vi "v2.62.vi"() -> ()   [LabVIEW 2018]
uses:
  <vilib>/DAQmx/read.llb/DAQmx Read (Analog 1D DBL NChan 1Samp).vi
  <extravilib>/ChannelInstances/High Speed Stream-c(a[.](c(dbl,dbl,dbl,dbl)),stamp,a[.](dbl),c(dbl,dbl,dbl,dbl,dbl,dbl,dbl))/_Read For Replicate.vi
  <extravilib>/ChannelInstances/High Speed Stream-c(a[.](c(dbl,dbl,dbl,dbl)),stamp,a[.](dbl),c(dbl,dbl,dbl,dbl,dbl,dbl,dbl))/Instantiate.vi
  <vilib>/Utility/file.llb/Write Delimited Spreadsheet (string).vi
  <extravilib>/ChannelInstances/High Speed Stream-c(a[.](c(dbl,dbl,dbl,dbl)),stamp,a[.](dbl),c(dbl,dbl,dbl,dbl,dbl,dbl,dbl))/)Channel.vi
  <extravilib>/ChannelInstances/High Speed Stream-c(a[.](c(dbl,dbl,dbl,dbl)),stamp,a[.](dbl),c(dbl,dbl,dbl,dbl,dbl,dbl,dbl))/Abort Signal/Init Signal.vi
  <vilib>/DAQmx/create/channels.llb/DAQmx Create Channel (AI-Temperature-Thermocouple).vi
  <vilib>/DAQmx/configure/timing.llb/DAQmx Timing (Sample Clock).vi
  <vilib>/DAQmx/miscellaneous.llb/DAQmx Fill In Error Info.vi
  <extravilib>/ChannelInstances/High Speed Stream-c(a[.](c(dbl,dbl,dbl,dbl)),stamp,a[.](dbl),c(dbl,dbl,dbl,dbl,dbl,dbl,dbl)).lvlib
panel:
  in  "file path (dialog if empty)":path
  out "Enum":T1(ring)
  in  "Start Recording?":bool
  in  "Stop Recording?":bool
  in  "Flowrate Control":dbl
  out "Status":T2(ring)
  in  "OK Button":bool
  in  "DAQ Properties":cluster{"Sample Rate":dbl}={"Sample Rate"=1.0} {"Sample Rate" min=0.1 max=10000.0 step=0.1}
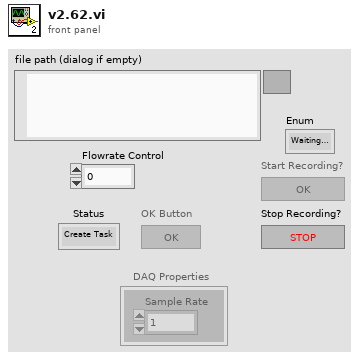
[diagram p1: front panel]
types:
  T1 = enum16{"Waiting to record", "Creating Spreadsheet", "Recording", "Finished Recording"}
  T2 = enum16{"Create Task", "Change Settings", "Check Settings", "Read Data", "End Task"}
  T3 = enum8{"Enabled", "Disabled", "Disabled and Grayed Out"}
  T4 = cluster{"Flowrate Data":cluster{"Line Number":dbl, "Temperature":dbl, "Pressure":dbl, "Flowrate":dbl}[], "Current Time":timestamp, "DAQmx Data":dbl[], "Rig Temperatures":cluster{"BRNR FC":dbl, "BRNR Nozzle":dbl, "Lance Tip":dbl, "Tube 2 Tmp":dbl, "Tube Tmp":dbl, "GA GAS Tmp":dbl, "Chamber External Temp":dbl}}
  T5 = cluster{"BRNR FC":dbl, "BRNR Nozzle":dbl, "Lance Tip":dbl, "Tube 2 Tmp":dbl, "Tube Tmp":dbl, "GA GAS Tmp":dbl, "Chamber External Temp":dbl}
  T6 = cluster{"Line Number":dbl, "Temperature":dbl, "Pressure":dbl, "Flowrate":dbl}[]
  T7 = typedef "High Speed Stream-c(a[.](c(dbl,dbl,dbl,dbl)),stamp,a[.](dbl),c(dbl,dbl,dbl,dbl,dbl,dbl,dbl)).lvlib/)Channel.ctl" = refnum<queue>
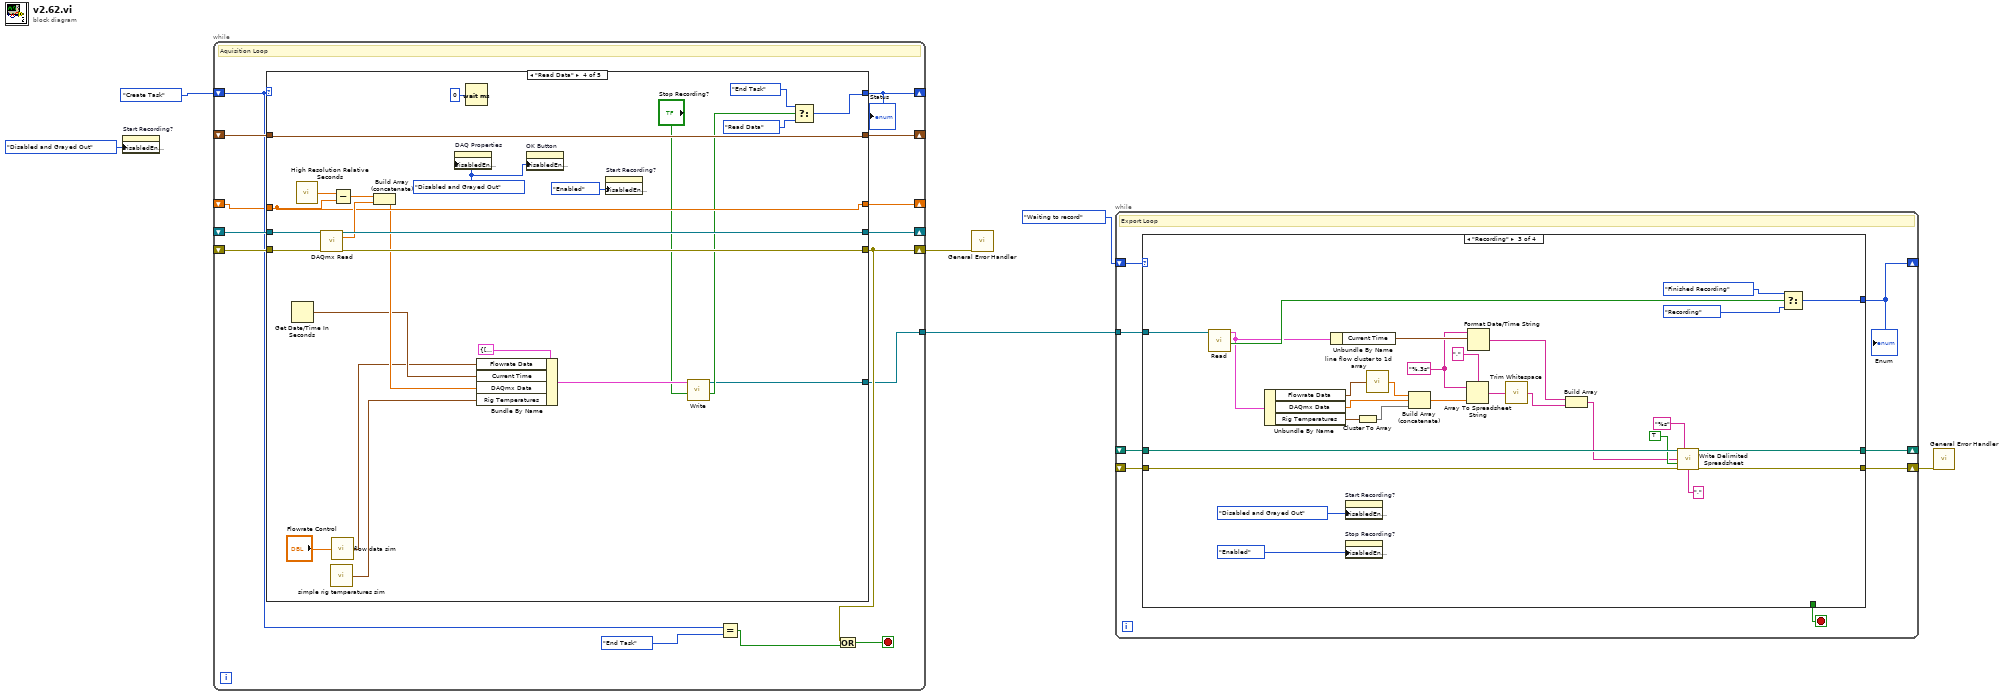
[diagram p0: block diagram]
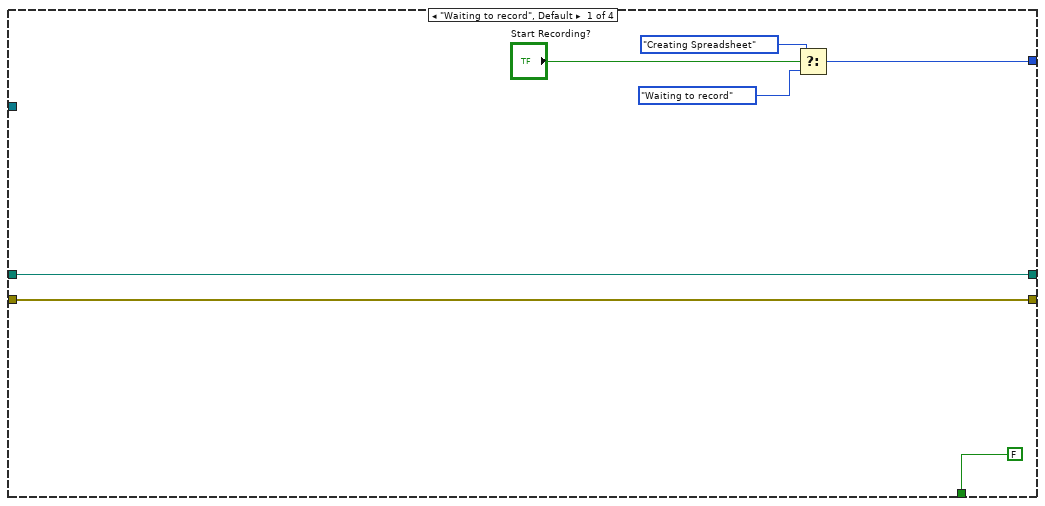
[diagram p2: hidden frame]
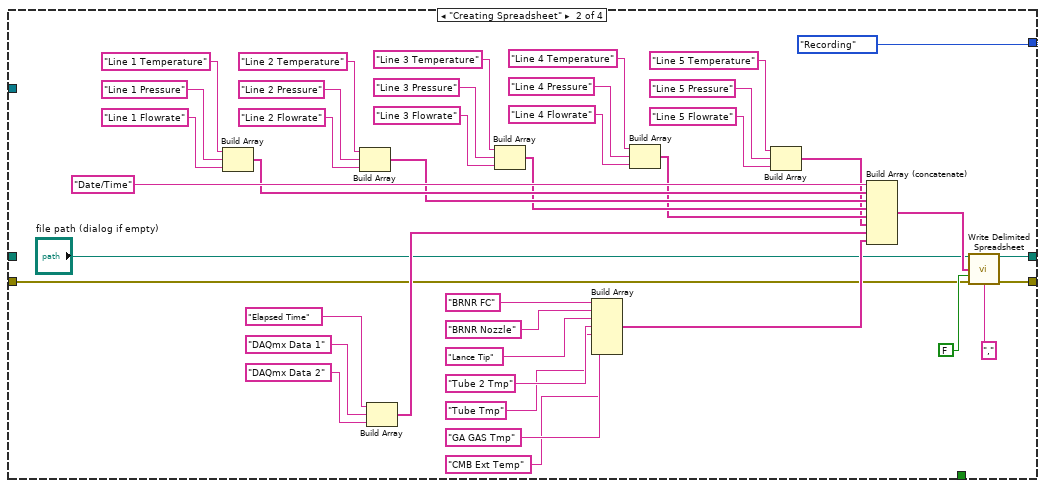
[diagram p3: hidden frame]
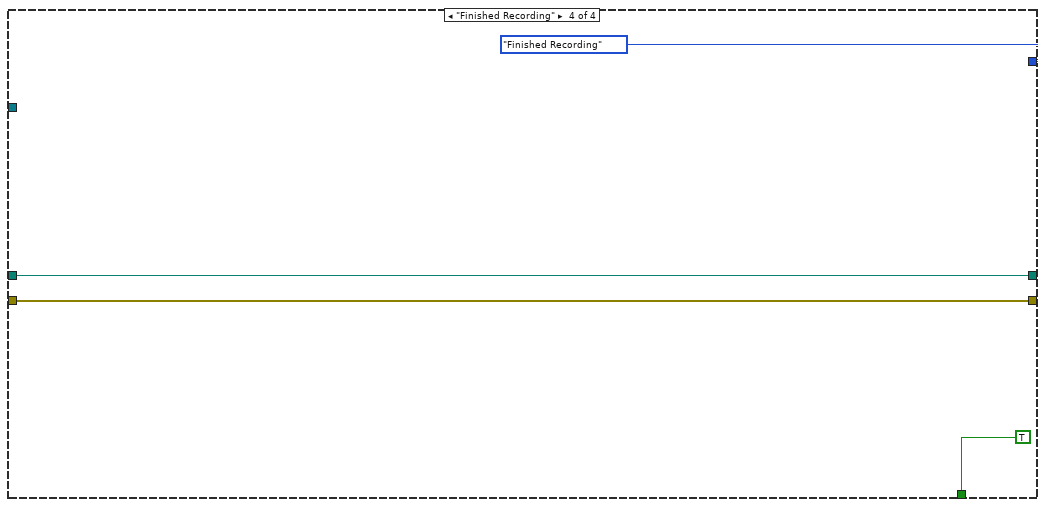
[diagram p4: hidden frame]
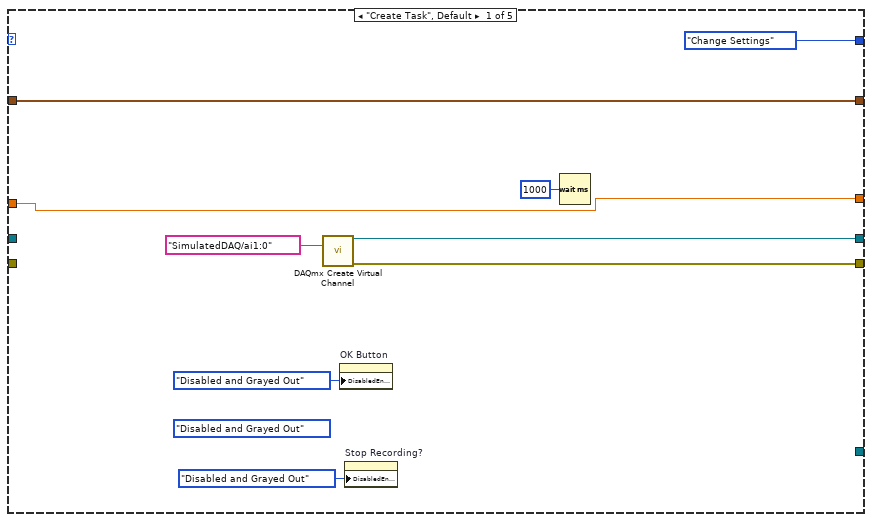
[diagram p5: hidden frame]
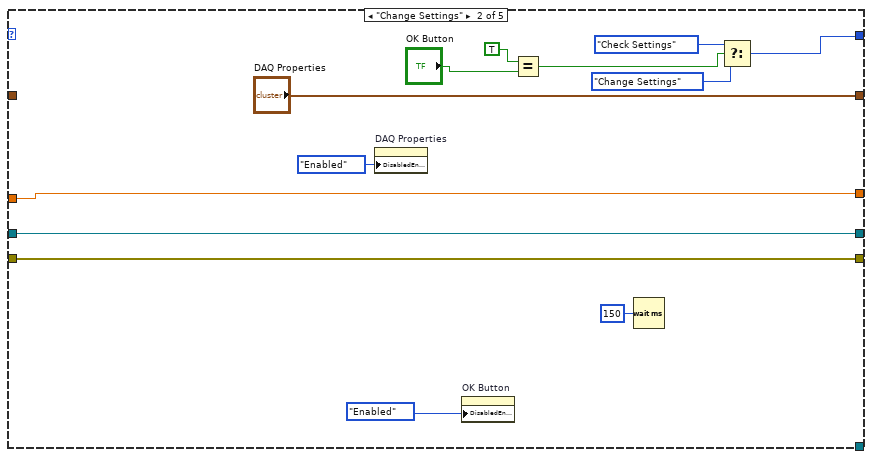
[diagram p6: hidden frame]
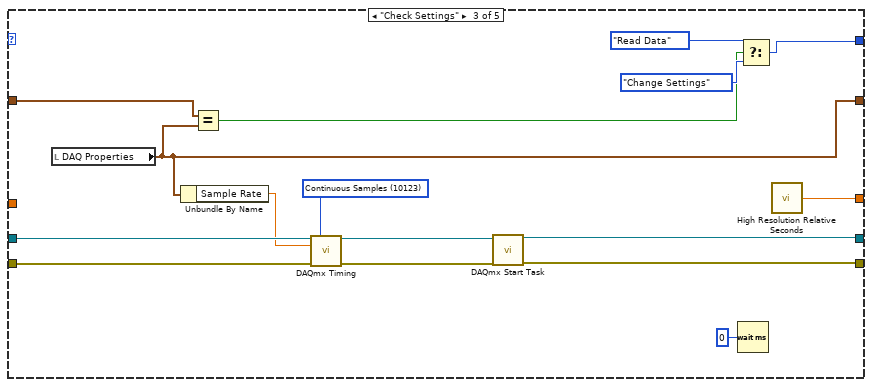
[diagram p7: hidden frame]
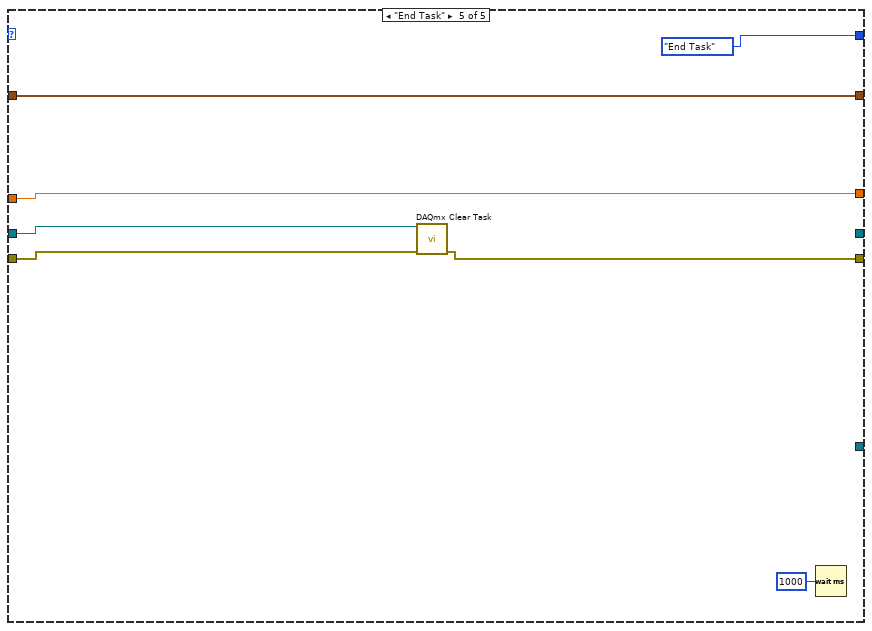
[diagram p8: hidden frame]
diagram:
  n1 = property on="Start Recording?" class="Bool"("DisabledEnum"=T3."Disabled and Grayed Out" ("Disabled")) -> ()  [unwired: 2 in, 2 out]
  n2 = while {
    shift-right: [w15] -> _
    shift-left: T2."Create Task" -> [w11]
    shift-right: [w20] -> _
    shift-left: _ -> [w18]
    shift-right: [w14] -> w2
    shift-left: _ -> [w17]
    shift-right: [w19] -> _
    shift-left: _ -> [w16]
    shift-right: [w10] -> _
    shift-left: _ -> [w9]
    tunnel: [w7] -> w4
    stop <- w8 stop-if-true
    # "Aquisition Loop"
    n3 = case shown="\"Read Data\"" w11 {
      tunnel: [w29 w42 w47 w80 _] -> w20
      tunnel: [w28 w41 w46 w79 w90] -> w14
      tunnel: [T2."Change Settings" w35 w54 w77 T2."End Task"] -> w15
      tunnel: [w25 "DAQ Properties" w50 w81 w89] -> w19
      tunnel: w18 -> [_ w42 w53 w83 w87]
      tunnel: w17 -> [_ w41 w52 w82 w86]
      tunnel: w16 -> [w25 _ w58 w81 w89]
      tunnel: [w23 w32 w43 w71 w85] -> w10
      tunnel: w9 -> [w23 w32 _ w71 w85]
      tunnel: [_ _ _ w61 _] -> w7
      frame "Create Task", Default {
        (unwired) T3."Disabled and Grayed Out" ("Disabled")
        n4 = call-poly <vilib>:"DAQmx Create Virtual Channel.vi"("physical channels"=tag "SimulatedDAQ/ai1:0") -> ("task out"=w29:refnum<k21>, "error out"=w28:errorcluster)  [unwired: 13 in]
        n5 = property on="OK Button" class="Bool"("DisabledEnum"=T3."Disabled and Grayed Out" ("Disabled")) -> ()  [unwired: 2 in, 2 out]
        n6 = property on="Stop Recording?" class="Bool"("DisabledEnum"=T3."Disabled and Grayed Out" ("Disabled")) -> ()  [unwired: 2 in, 2 out]
        n7 = Wait (ms)(milliseconds to wait=u32 1000) -> ()  [unwired: 1 out]
      }
      frame "Change Settings" {
        n8 = property on="DAQ Properties" class="Clust (strict)"("DisabledEnum"=T3."Enabled" ("Disabled")) -> ()  [unwired: 2 in, 2 out]
        n9 = property on="OK Button" class="Bool"("DisabledEnum"=T3."Enabled" ("Disabled")) -> ()  [unwired: 2 in, 2 out]
        n10 = Equal?(x=TRUE, y="OK Button") -> (x = y?=w37:bool)
        n11 = Wait (ms)(milliseconds to wait=u32 150) -> ()  [unwired: 1 out]
        n12 = Select(t=T2."Check Settings", s=w37, f=T2."Change Settings") -> (s? t:f=w35:T2)
      }
      frame "Check Settings" {
        w44 = 10123 items=["Finite Samples"=10178, "Continuous Samples"=10123, "Hardware Timed Single Point"=12522] ("sample mode")
        n13 = local read "DAQ Properties"() -> (w50:cluster{"Sample Rate":dbl})
        n14 = Unbundle By Name(w50) -> ("Sample Rate"=w51:dbl)
        n15 = Equal?(x=w58, y=w50) -> (x = y?=w45:bool)
        n16 = call-poly <vilib>:"DAQmx Timing.vi"("task/channels in"=w53, "sample mode"=w44, "rate"=w51, "error in"=w52) -> ("task out"=w49:refnum<k21>, "error out"=w48:errorcluster)  [unwired: 10 in]
        n17 = call <vilib>:"DAQmx Start Task.vi"("task/channels in"=w49, "error in"=w48) -> ("task out"=w47:refnum<k21>, "error out"=w46:errorcluster)  [unwired: 12 in]
        n18 = Wait (ms)(milliseconds to wait=u32 0) -> ()  [unwired: 1 out]
        n19 = Select(t=T2."Read Data", s=w45, f=T2."Change Settings") -> (s? t:f=w54:T2)
        n20 = call <vilib>:"High Resolution Relative Seconds.vi"() -> ("relative seconds"=w43:dbl)
      }
      frame "Read Data" {
        w60 = T3."Disabled and Grayed Out" ("Disabled")
        n21 = Get Date/Time In Seconds() -> (seconds since 1Jan1904=w67:timestamp)
        n22 = call <vilib>:"High Resolution Relative Seconds.vi"() -> ("relative seconds"=w74:dbl)
        n23 = call-poly <vilib>:"DAQmx Read.vi"("task/channels in"=w83, "error in"=w82) -> ("task out"=w80:refnum<k21>, "data"=w73:dbl[], "error out"=w79:errorcluster)  [unwired: 11 in]
        n24 = call "simple rig temperatures sim.vi"() -> ("Rig Temperatures"=w65:T5)
        n25 = call "flow data sim.vi"("Boondoggle Input"="Flowrate Control") -> ("Flowrate Data"=w66:T6)
        n26 = Subtract(x=w74, y=w71) -> (x-y=w72:dbl)
        n27 = Build Array (concatenate)(w72, w73) -> (w68:dbl[])
        n28 = property on="DAQ Properties" class="Clust (strict)"("DisabledEnum"=w60) -> ()  [unwired: 2 in, 2 out]
        n29 = Wait (ms)(milliseconds to wait=u32 0) -> ()  [unwired: 1 out]
        n30 = Bundle By Name(cluster=T4 {"Flowrate Data"=[{"Line Number"=1.0, "Temperature"=17.480721541683437, "Pressure"=24.0, "Flowrate"=0.0}, {"Line Number"=2.0, "Temperature"=21.850901927104296, "Pressure"=30.0, "Flowrate"=0.0}, {"Line Number"=3.0, "Temperature"=26.221082312525155, "Pressure"=36.0, "Flowrate"=0.0}, {"Line Number"=4.0, "Temperature"=30.591262697946018, "Pressure"=42.00000000000001, "Flowrate"=0.0}, {"Line Number"=5.0, "Temperature"=34.96144308336687, "Pressure"=48.0, "Flowrate"=0.0}], "Current Time"=timestamp(0 s since 1904-01-01), "DAQmx Data"=[], "Rig Temperatures"={"BRNR FC"=0.0, "BRNR Nozzle"=0.0, "Lance Tip"=0.0, "Tube 2 Tmp"=0.0, "Tube Tmp"=0.0, "GA GAS Tmp"=0.0, "Chamber External Temp"=0.0}}, "Flowrate Data"=w66, "Current Time"=w67, "DAQmx Data"=w68, "Rig Temperatures"=w65) -> (w64:T4)
        n31 = property on="OK Button" class="Bool"("DisabledEnum"=w60) -> ()  [unwired: 2 in, 2 out]
        n32 = property on="Start Recording?" class="Bool"("DisabledEnum"=T3."Enabled" ("Disabled")) -> ()  [unwired: 2 in, 2 out]
        n33 = call <extravilib>:"Write.vi"("last element? (F)"="Stop Recording?", "element"=w64) -> ("done?"=w62:bool, "channel"=w61:T7)  [unwired: 7 in, 1 out]
        n34 = Select(t=T2."End Task", s=w62, f=T2."Read Data") -> (s? t:f=w77:T2)
      }
      frame "End Task" {
        n35 = call <vilib>:"DAQmx Clear Task.vi"("task in"=w87, "error in"=w86) -> ("error out"=w90:errorcluster)  [unwired: 13 in]
        n36 = Wait (ms)(milliseconds to wait=u32 1000) -> ()  [unwired: 1 out]
      }
    }
    "Status" <- w15
    n37 = Equal?(x=w11, y=T2."End Task") -> (x = y?=w12:bool)
    n38 = Or(x=w14, y=w12) -> (x .or. y?=w8:bool)
  }
  n39 = call <vilib>:"General Error Handler.vi"("error in (no error)"=w2) -> ()  [unwired: 10 in, 5 out]
  n40 = while {
    shift-right: [w98] -> _
    shift-left: T1."Waiting to record" -> [w97]
    tunnel: w4 -> [w95]
    shift-right: [w93] -> _
    shift-left: _ -> [w94]
    shift-right: [w92] -> w3
    shift-left: _ -> [w91]
    stop <- w96 stop-if-true
    # "Export Loop"
    n41 = case shown="\"Recording\"" w97 {
      tunnel: [w102 T1."Recording" w173 T1."Finished Recording"] -> w98
      tunnel: [FALSE _ _ TRUE] -> w96
      tunnel: w95 -> [_ _ w169 _]
      tunnel: w94 -> [w100 _ w166 w176]
      tunnel: [w100 w125 w167 w176] -> w93
      tunnel: [w99 w107 w156 w175] -> w92
      tunnel: w91 -> [w99 w108 w155 w175]
      frame "Waiting to record", Default {
        n42 = Select(t=T1."Creating Spreadsheet", s="Start Recording?", f=T1."Waiting to record") -> (s? t:f=w102:T1)
      }
      frame "Creating Spreadsheet" {
        n43 = Build Array("Line 1 Temperature", "Line 1 Pressure", "Line 1 Flowrate") -> (w130:string[])
        n44 = Build Array("Line 2 Temperature", "Line 2 Pressure", "Line 2 Flowrate") -> (w129:string[])
        n45 = Build Array("Elapsed Time", "DAQmx Data 1", "DAQmx Data 2") -> (w118:string[])
        n46 = Build Array("Line 3 Temperature", "Line 3 Pressure", "Line 3 Flowrate") -> (w128:string[])
        n47 = Build Array("BRNR FC", "BRNR Nozzle", "Lance Tip", "Tube 2 Tmp", "Tube Tmp", "GA GAS Tmp", "CMB Ext Temp") -> (w110:string[])
        n48 = Build Array("Line 4 Temperature", "Line 4 Pressure", "Line 4 Flowrate") -> (w127:string[])
        n49 = Build Array("Line 5 Temperature", "Line 5 Pressure", "Line 5 Flowrate") -> (w119:string[])
        n50 = Build Array (concatenate)("Date/Time", w130, w129, w128, w127, w119, w118, w110) -> (w124:string[])
        n51 = call-poly <vilib>:"Write Delimited Spreadsheet.vi"("file path (dialog if empty)"="file path (dialog if empty)", "1D data"=w124, "append to file? (new file:F)"=FALSE, "error in (no error)"=w108, "delimiter (\\t)"="," ("delimiter (\\t)")) -> ("new file path (Not A Path if cancelled)"=w125:path, "error out"=w107:errorcluster)  [unwired: 9 in]
      }
      frame "Recording" {
        w147 = "%.3s" ("format string")
        n52 = call <extravilib>:"Read.vi"("channel"=w169) -> ("done?"=w168:bool, "element"=w163:T4)  [unwired: 6 in, 3 out]
        n53 = Unbundle By Name(w163) -> ("Flowrate Data"=w164:T6, "DAQmx Data"=w160:dbl[], "Rig Temperatures"=w170:T5)
        n54 = Unbundle By Name(w163) -> ("Current Time"=w162:timestamp)
        n55 = property on="Start Recording?" class="Bool"("DisabledEnum"=T3."Disabled and Grayed Out" ("Disabled")) -> ()  [unwired: 2 in, 2 out]
        n56 = property on="Stop Recording?" class="Bool"("DisabledEnum"=T3."Enabled" ("Disabled")) -> ()  [unwired: 2 in, 2 out]
        n57 = Cluster To Array(cluster=w170) -> (array=w161:dbl[])
        n58 = call "line flow cluster to 1d array.vi"("Flowrate Data"=w164) -> ("Array"=w159:dbl[])
        n59 = Build Array (concatenate)(w159, w160, w161) -> (w158:dbl[])
        n60 = Array To Spreadsheet String(delimiter (Tab)=",", array=w158, 3:w147) -> (spreadsheet string=w150:string)
        n61 = Format Date/Time String(time format string (%c)=w147, seconds (now)=w162) -> (date/time string=w151:string)  [unwired: 1 in]
        n62 = call <vilib>:"Trim Whitespace.vi"("string"=w150) -> ("trimmed string"=w149:string)  [unwired: 1 in]
        n63 = Build Array(w151, w149) -> (w152:string[])
        n64 = call-poly <vilib>:"Write Delimited Spreadsheet.vi"("file path (dialog if empty)"=w166, "format (%s)"="%s", "1D data"=w152, "append to file? (new file:F)"=TRUE, "error in (no error)"=w155, "delimiter (\\t)"="," ("delimiter (\\t)")) -> ("new file path (Not A Path if cancelled)"=w167:path, "error out"=w156:errorcluster)  [unwired: 8 in]
        n65 = Select(t=T1."Finished Recording", s=w168, f=T1."Recording") -> (s? t:f=w173:T1)
      }
      frame "Finished Recording" {
      }
    }
    "Enum" <- w98
  }
  n66 = call <vilib>:"General Error Handler.vi"("error in (no error)"=w3) -> ()  [unwired: 10 in, 5 out]
